vi "HexapodInitializeHardware.vi"(8 "error in (no error)":errorcluster) -> (0 "error out":errorcluster, 2 "devaddress":string)   [LabVIEW 2020]
uses:
  <vilib>/Instr/_visa.llb/VISA Configure Serial Port (Instr).vi
  C-887.lvclass
  C:/GEECS/Developers Version/source/Device Drivers/HexapodPI/HexapodPI.lvclass
  C:/GEECS/Developers Version/source/Device Drivers/BaseDriver/BaseDriver.lvclass
  C:/GEECS/Developers Version/source/Device Drivers/HexapodPI/C-887_Driver/C-887.lvclass
panel:
  out "C-887 out":refnum<class "C-887.lvclass">
  in  "C-887 in":refnum<class "C-887.lvclass">
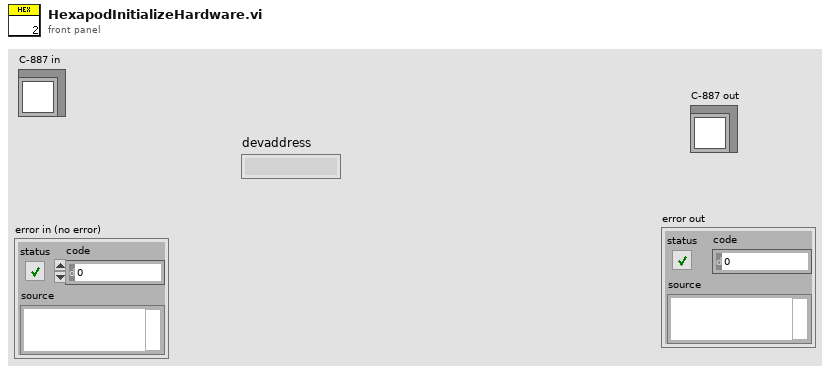
[diagram p1: front panel]
types:
  T1 = cluster{"connection ID":refnum<k5>, "VISA resource name out":refnum<visa-resource-name>, "connectiontype":void}
  T2 = cluster{"connection ID":refnum<k5>, "VISA resource name":refnum<visa-resource-name>, "Selector":enum16{"TCPIP", "Serial"}}
  T3 = cluster{"connection ID":refnum<k5>, "VISA Refnum out":refnum<visa-resource-name>, "Selector":enum16{"TCPIP", "Serial"}}
  T4 = cluster{"Strut 1 motion error":bool, "Strut 2 motion error":bool, "Strut 3 motion error":bool, "Strut 4 motion error":bool, "Strut 5 motion error":bool, "Strut 6 motion error":bool, "Axis A motion error":bool, "Axis B motion error":bool, "Strut 1 in motion":bool, "Strut 2 in motion":bool, "Strut 3 in motion":bool, "Strut 4 in motion":bool, "Strut 5 in motion":bool, "Strut 6 in motion":bool, "Axis A in motion":bool, "Axis B in motion":bool, "Hexapod is Initialized":bool, "Stage A is Initialized":bool, "Stage B is Initialized":bool, "Initialisation in progress":bool}
  T5 = typedef "PivotPoint_TypDef.ctl" = cluster{"R":cluster{"Value":dbl, "Min":dbl, "Max":dbl, "StepSize":dbl, "Tolerance":dbl, "ValueActual":dbl}, "S":cluster{"Value":dbl, "Min":dbl, "Max":dbl, "StepSize":dbl, "Tolerance":dbl, "ValueActual":dbl}, "T":cluster{"Value":dbl, "Min":dbl, "Max":dbl, "StepSize":dbl, "Tolerance":dbl, "ValueActual":dbl}}
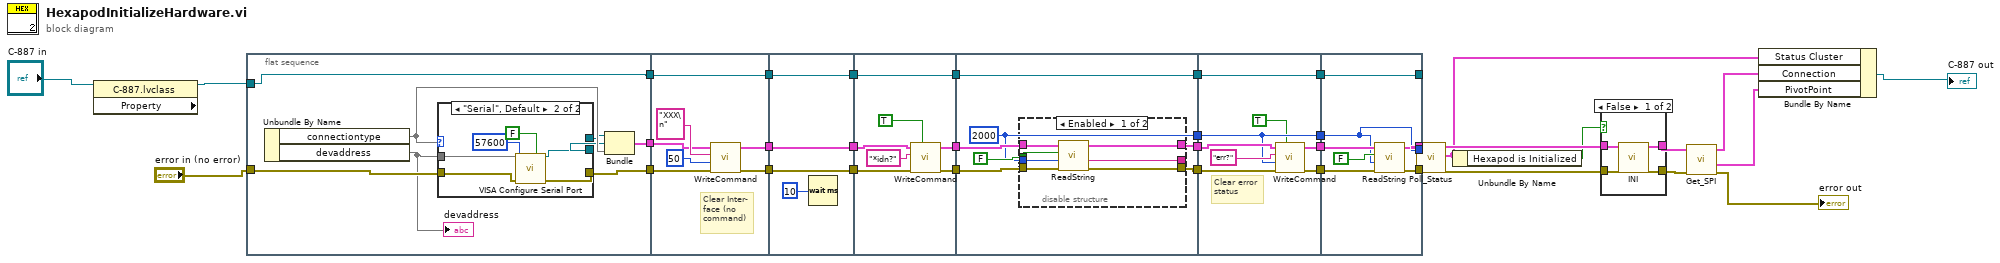
[diagram p0: block diagram]
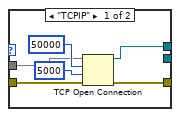
[diagram p3: hidden frame]
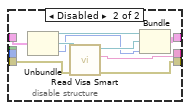
[diagram p4: hidden frame]
diagram:
  n1 = property class="C-887.lvclass" props=[](reference="C-887 in") -> (reference out=w3:refnum<class "C-887.lvclass">)  [unwired: 1 in, 2 out]
  n2 = flat-sequence {
    tunnel: "error in (no error)" -> [w46]
    tunnel: [w45] -> w37
    tunnel: [w42] -> w36
    tunnel: w3 -> [w38]
    tunnel: [w38] -> w14
    tunnel: [w64] -> w35
    tunnel: [w62] -> w34
    tunnel: w37 -> [w63]
    tunnel: w36 -> [w60]
    tunnel: w14 -> [w59]
    tunnel: [w59] -> w11
    tunnel: w35 -> [w68]
    tunnel: [w68] -> w33
    tunnel: [w67] -> w32
    tunnel: w34 -> [w67]
    tunnel: [w66] -> w12
    tunnel: w11 -> [w66]
    tunnel: w33 -> [w76]
    tunnel: [w71] -> w31
    tunnel: w32 -> [w74]
    tunnel: [w73] -> w30
    tunnel: [w70] -> w13
    tunnel: w12 -> [w70]
    tunnel: w31 -> [w83]
    tunnel: [w78] -> w29
    tunnel: w30 -> [w81]
    tunnel: [w80] -> w28
    tunnel: [w79] -> w27
    tunnel: w13 -> [w77]
    tunnel: [w77] -> w9
    tunnel: w29 -> [w107]
    tunnel: [w106] -> w26
    tunnel: w28 -> [w103]
    tunnel: [w104] -> w25
    tunnel: w27 -> [w102]
    tunnel: [w102] -> w24
    tunnel: [w100] -> w10
    tunnel: w9 -> [w100]
    tunnel: w26 -> [w114]
    tunnel: [w113] -> w16
    tunnel: w25 -> [w111]
    tunnel: [w110] -> w15
    tunnel: w24 -> [w109]
    tunnel: [w109] -> w20
    tunnel: [w108] -> w8
    tunnel: w10 -> [w108]
    frame #0 {
      n3 = Unbundle By Name() -> (w39:refnum<class "C-887.lvclass">, "connectiontype"=w43, "devaddress"=w44)
      "devaddress" <- w44
      n4 = case shown="\"Serial\", Default" w43 {
        tunnel: w46 -> [w50 w54]
        tunnel: [w49 w57] -> w45
        tunnel: [w48 _] -> w40
        tunnel: w44 -> [w47 w55]
        tunnel: [_ w58] -> w41
        frame "TCPIP" {
          n5 = TCP Open Connection(address=w47, remote port or service name=u16 50000, timeout ms (60000)=5000, error in (no error)=w50) -> (connection ID=w48:refnum<k5>, error out=w49:errorcluster)  [unwired: 1 in]
        }
        frame "Serial", Default {
          n6 = call-poly "VISA Configure Serial Port"("VISA resource name"=w55, "Enable Termination\nChar (T)"=FALSE ("Enable Termination\nChar (T)"), "baud rate (9600)"=u32 57600, "error in (no error)"=w54) -> ("VISA resource name out"=w58:refnum<visa-resource-name>, "error out"=w57:errorcluster)  [unwired: 10 in]
        }
      }
      n7 = Bundle("connection ID"=w40, "VISA resource name out"=w41, "connectiontype"=w43) -> (w42:T1)  [unwired: 1 in]
    }
    frame #1 {
      # "Clear Inter-\nface (no\ncommand)"
      n8 = call "WriteCommand.vi"("error in (no error)"=w63, "timeout ms (0)"=50, "String"="XXX\n" ("Interface clear"), "Connection"=w60) -> ("error out"=w64:errorcluster, "Connection out"=w62:T2)  [unwired: 6 in]
    }
    frame #2 {
      n9 = Wait (ms)(milliseconds to wait=u32 10) -> ()  [unwired: 1 out]
    }
    frame #3 {
      n10 = call "WriteCommand.vi"("Attach Linefeed"=TRUE, "error in (no error)"=w76, "String"="*idn?" ("String to Send"), "Connection"=w74) -> ("error out"=w71:errorcluster, "Connection out"=w73:T2)  [unwired: 6 in]
    }
    frame #4 {
      w79 = 2000 ("timeout ms (0)")
      n11 = disable-structure shown="Enabled" {
        disable-tunnel: w83 -> [w90 w98]
        disable-tunnel: [w89 w91] -> _
        disable-tunnel: FALSE ("Strip spaces?") -> [w88 _]
        disable-tunnel: w81 -> [w87 w97]
        disable-tunnel: [w86 w94] -> w80
        disable-tunnel: w79 -> [w85 _]
        disable-tunnel: [w84 w99] -> w78
        frame Enabled {
          n12 = call "ReadString.vi"("error in (no error)"=w90, "timeout ms (0)"=w85, "Trim Spaces"=w88, "Connection"=w87) -> ("error out"=w84:errorcluster, "String out"=w89:string, "Connection out"=w86:T2)  [unwired: 5 in]
        }
        frame Disabled {
          n13 = Unbundle(w97) -> ("connection ID"=w95:refnum<k5>, "VISA resource name"=w96:refnum<visa-resource-name>, "Selector"=w92:enum16{"TCPIP", "Serial"})
          n14 = call "Read Visa Smart.vi"("error in (no error)"=w98, "VISA Refnum in"=w96) -> ("error out"=w99:errorcluster, "String"=w91:string, "VISA Refnum out"=w93:refnum<visa-resource-name>)  [unwired: 7 in]
          n15 = Bundle("connection ID"=w95, "VISA Refnum out"=w93, "Selector"=w92) -> (w94:T3)  [unwired: 1 in]
        }
      }
    }
    frame #5 {
      # "Clear error\nstatus"
      n16 = call "WriteCommand.vi"("Attach Linefeed"=TRUE, "error in (no error)"=w107, "timeout ms (0)"=w102, "String"="err?" ("String to Send"), "Connection"=w103) -> ("error out"=w106:errorcluster, "Connection out"=w104:T2)  [unwired: 5 in]
    }
    frame #6 {
      n17 = call "ReadString.vi"("error in (no error)"=w114, "timeout ms (0)"=w109, "Trim Spaces"=FALSE ("Strip spaces?"), "Connection"=w111) -> ("error out"=w113:errorcluster, "Connection out"=w110:T2)  [unwired: 5 in, 1 out]
    }
  }
  n18 = call "Poll_Status.vi"("Connection"=w15, "timeout ms (0)"=w20, "error in"=w16) -> ("Connection out"=w18:T2, "Status Cluster"=w7:T4, "error out"=w19:errorcluster)  [unwired: 14 in]
  n19 = Unbundle By Name(w7) -> ("Hexapod is Initialized"=w17:bool)
  n20 = case shown="False" w17 {
    tunnel: w18 -> [w118 w120]
    tunnel: [w117 w120] -> w21
    tunnel: w19 -> [w116 w119]
    tunnel: [w115 w119] -> w22
    frame False {
      n21 = call "INI.vi"("Connection"=w118, "error in"=w116) -> ("Connection out"=w117:T2, "error out"=w115:errorcluster)  [unwired: 16 in]
    }
    frame True {
    }
  }
  n22 = call "Get_SPI.vi"("error in (no error)"=w22, "Connection"=w21) -> ("error out"=→"error out":errorcluster, "PivotPoint"=w5:T5, "Connection out"=w6:T2)  [unwired: 6 in, 1 out]
  n23 = Bundle By Name("Status Cluster"=w7, "Connection"=w6, "PivotPoint"=w5) -> (→"C-887 out":refnum<class "C-887.lvclass">)  [unwired: 1 in]
